vi "UT_TCP2Foxconn.vi"() -> ()   [LabVIEW 2019, in "TCP2Foxconn.lvlib"]
uses:
  TCP2Foxconn.lvlib
panel:
  in  "One shot Second HandShake":bool
  in  "One shot First HandShake":bool
  out "Second Handshake Response":string="NG;;ORA-06502: PL/SQL: numeric or value error: character to number conversion error\nORA-06512: at \"SFIS1.LASER_CARVING_AA\", line 34\n;SN:TKSR131A1T2222000031,OK,LASEREND;"
  out "First Handshake Response":string
  in  "Second HandShake":bool
  in  "First HandShake":bool
  in  "Result":string="OK"
  in  "Barcode":string="TKSR131A1T2222000031"
  out "Error Out":errorcluster
  in  "Error In":errorcluster
  in  "Close API":bool
  out "TCP connected":bool
  in  "Close Connection":bool
  in  "Open Connection":bool
  in  "IP address":string="10.61.39.233:60003"
  # "2111170002800000320754"
  # "TKSR131A1T2222000019"
  # "TKSR131A1T2222000031"
  # "TKSR131A1T2222000040"
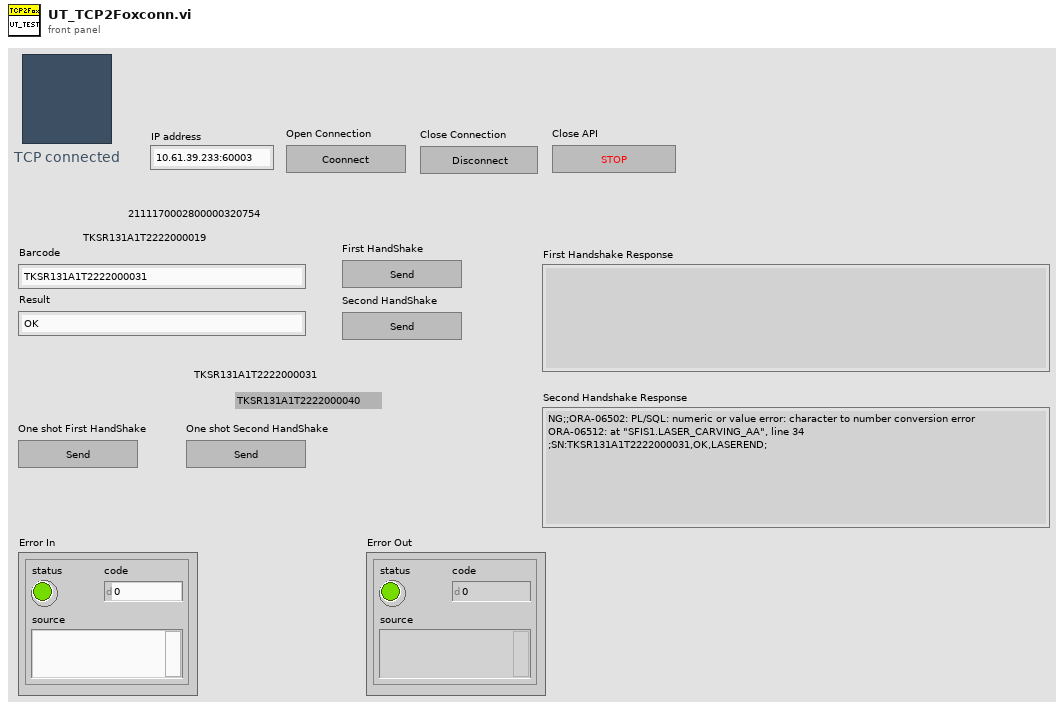
[diagram p1: front panel]
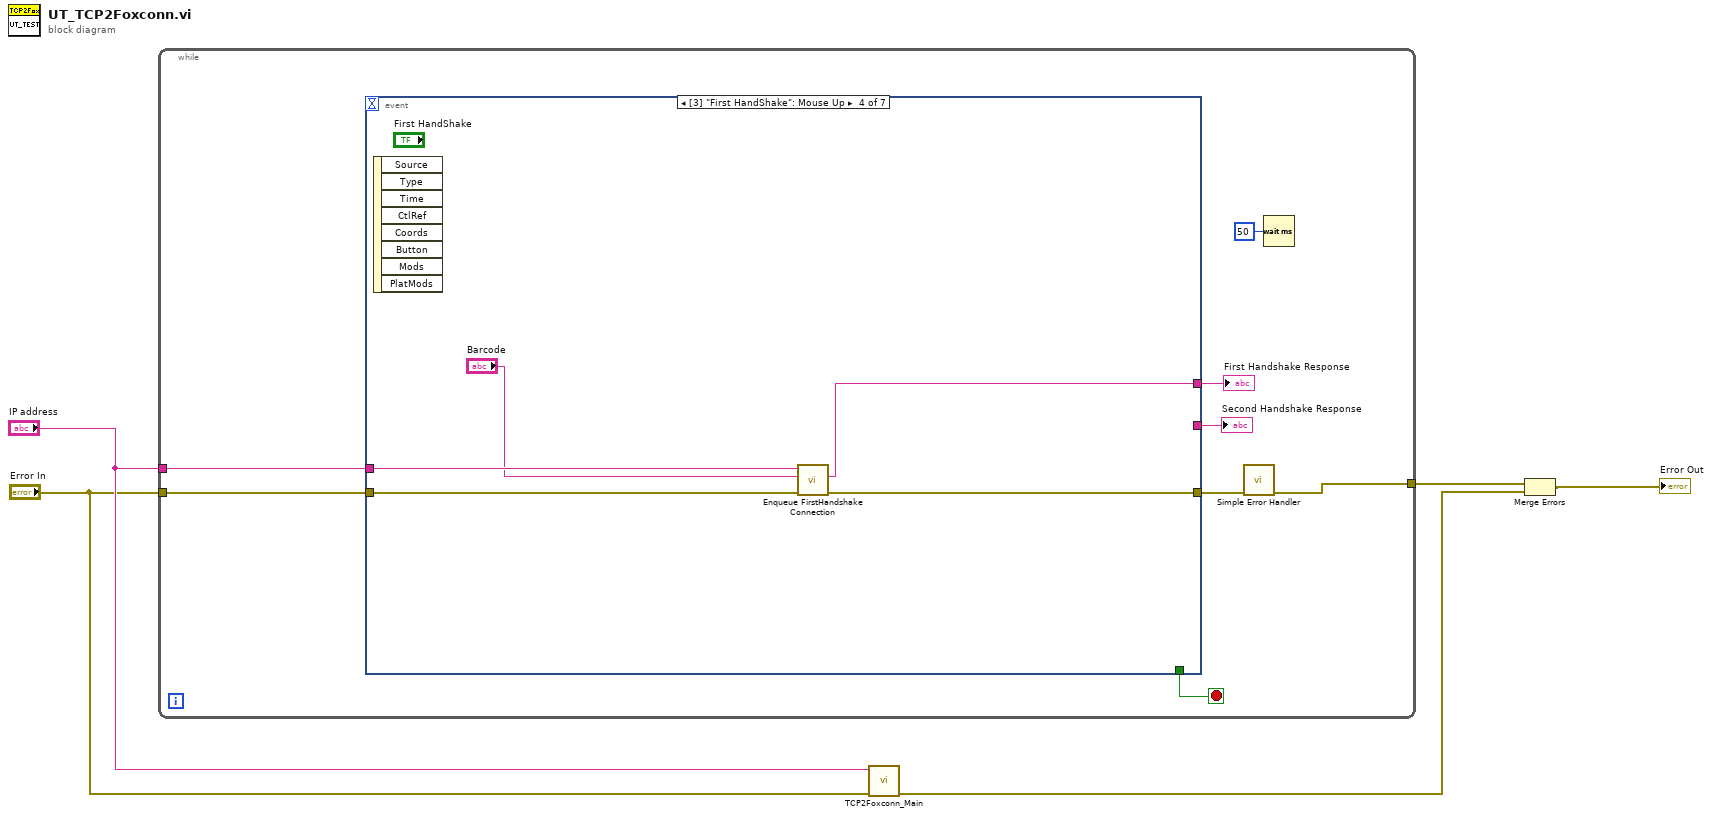
[diagram p0: block diagram]
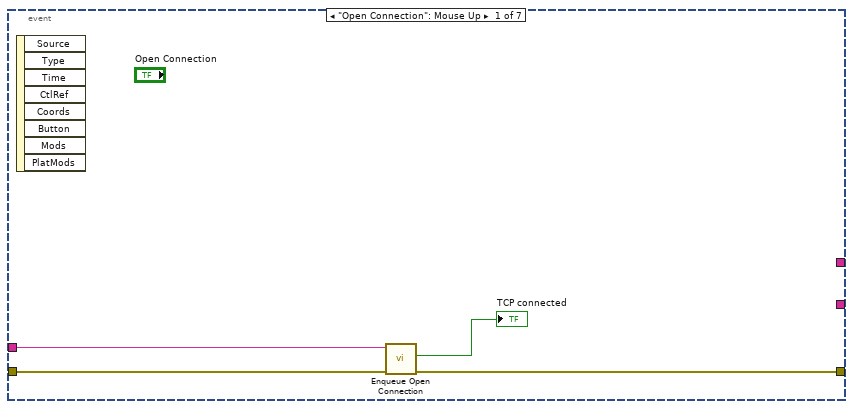
[diagram p2: hidden frame]
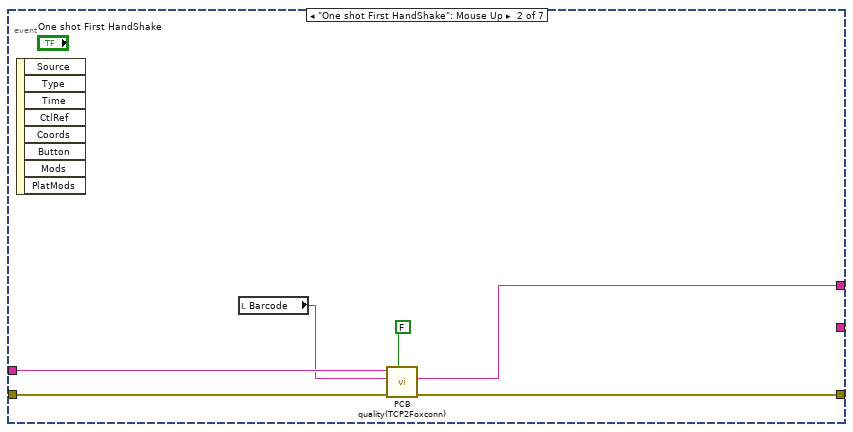
[diagram p3: hidden frame]
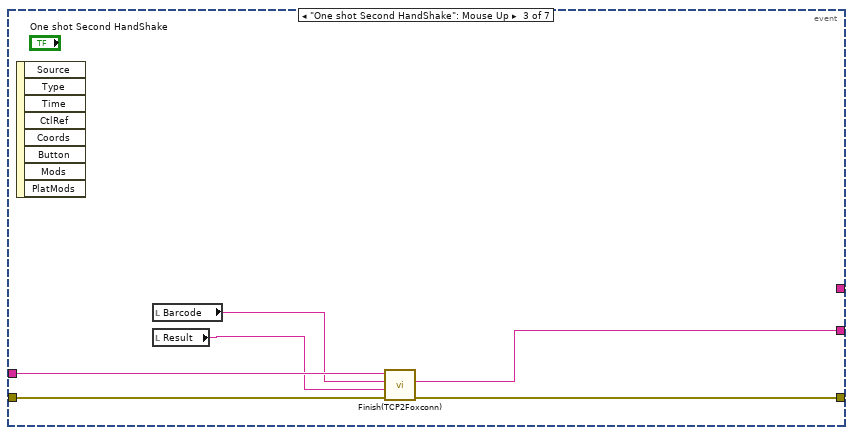
[diagram p4: hidden frame]
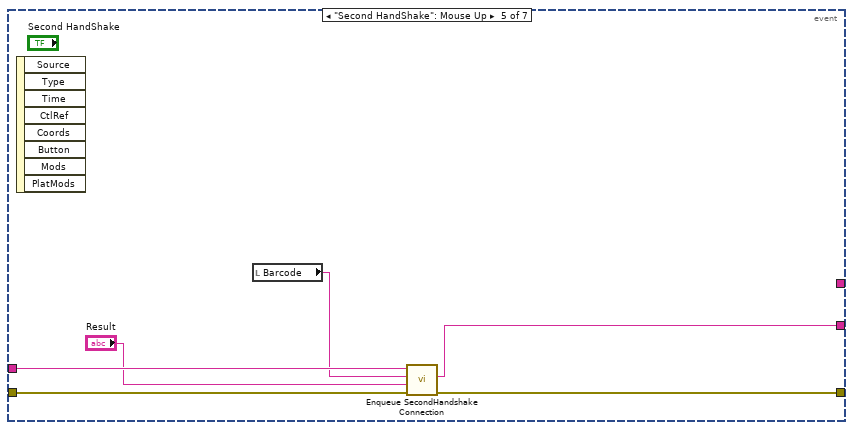
[diagram p5: hidden frame]
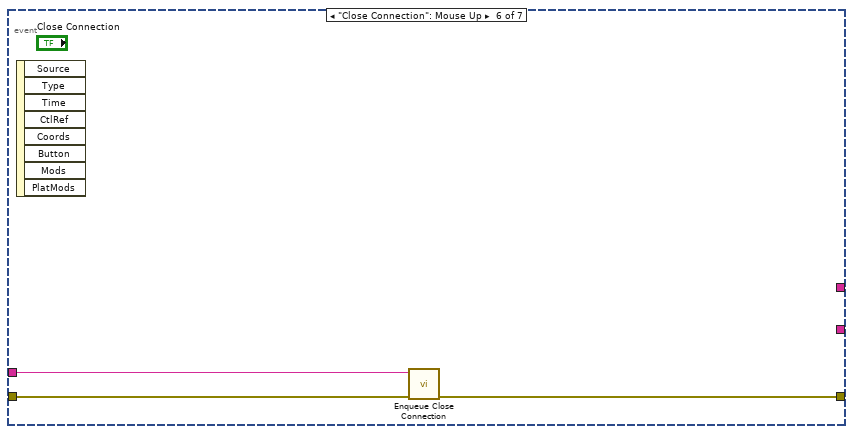
[diagram p6: hidden frame]
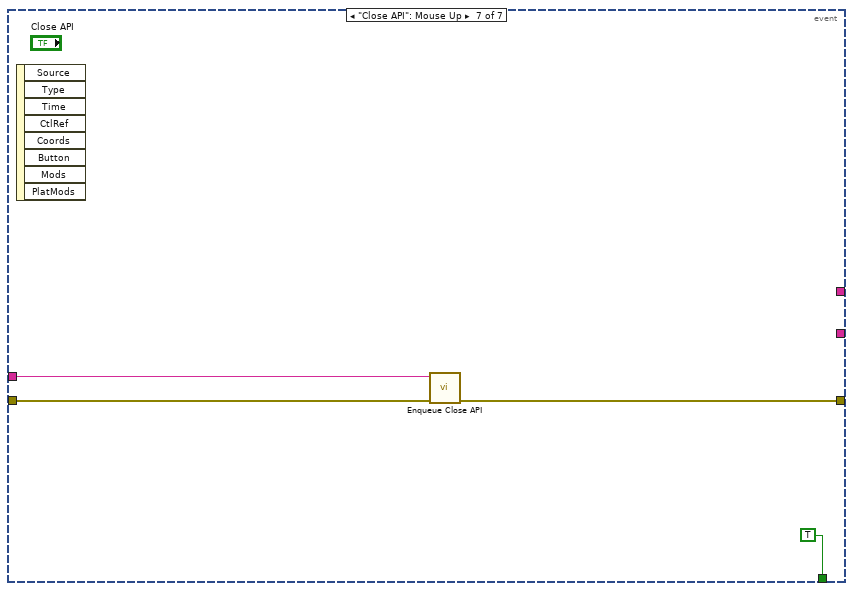
[diagram p7: hidden frame]
diagram:
  n1 = while {
    tunnel: "IP address" -> [w13]
    tunnel: "Error In" -> [w12]
    tunnel: [w10] -> w3
    stop <- w8 stop-if-true
    n2 = event shown="[3] \"First HandShake\": Mouse Up" {
      selector: _ -> [_ _ _ _ _ _ _]
      dyn-events: _ -> [_ _ _ _ _ _ _]
      timeout: _ -> [_ _ _ _ _ _ _]
      tunnel: w13 -> [w17 w23 w29 w34 w38 w41 w45]
      tunnel: w12 -> [w16 w22 w28 w33 w40 w43 w47]
      tunnel: [w15 w20 w24 w32 w39 w42 w46] -> w11
      tunnel: [_ _ _ _ _ _ TRUE] -> w8
      tunnel: [_ w21 _ w31 _ _ _] -> w7
      tunnel: [_ _ w25 _ w35 _ _] -> w6
      event "Open Connection": Mouse Up {
        n3 = event-data() -> ()  [unwired: 1 in, 8 out]
        n4 = call "Enqueue Open Connection.vi"("Error In"=w16, "Name"=w17) -> ("Error Out"=w15:errorcluster, "Connect?"=→"TCP connected":bool)  [unwired: 8 in]
      }
      event "One shot First HandShake": Mouse Up {
        n5 = event-data() -> ()  [unwired: 1 in, 8 out]
        n6 = local read "Barcode"() -> (w18:string)
        n7 = call "PCB quality(TCP2Foxconn).vi"("Bypass查詢"=FALSE, "error in (no error)"=w22, "Barcode"=w18, "TCP2Foxc"=w23) -> ("error out"=w20:errorcluster, "result"=w21:string)  [unwired: 6 in]
      }
      event "One shot Second HandShake": Mouse Up {
        n8 = event-data() -> ()  [unwired: 1 in, 8 out]
        n9 = local read "Barcode"() -> (w27:string)
        n10 = local read "Result"() -> (w26:string)
        n11 = call "Finish(TCP2Foxconn).vi"("error in (no error)"=w28, "Result"=w26, "Barcode"=w27, "TCP2Foxc"=w29) -> ("error out"=w24:errorcluster, "result"=w25:string)  [unwired: 6 in]
      }
      event "First HandShake": Mouse Up {
        n12 = event-data() -> ()  [unwired: 1 in, 8 out]
        n13 = call "Enqueue FirstHandshake Connection.vi"("Error In"=w33, "Barcode"="Barcode", "Name"=w34) -> ("Error Out"=w32:errorcluster, "Result"=w31:string)  [unwired: 7 in]
      }
      event "Second HandShake": Mouse Up {
        n14 = event-data() -> ()  [unwired: 1 in, 8 out]
        n15 = local read "Barcode"() -> (w36:string)
        n16 = call "Enqueue SecondHandshake Connection.vi"("Error In"=w40, "Result"="Result", "Barcode"=w36, "Name"=w38) -> ("Error Out"=w39:errorcluster, "Result"=w35:string)  [unwired: 6 in]
      }
      event "Close Connection": Mouse Up {
        n17 = event-data() -> ()  [unwired: 1 in, 8 out]
        n18 = call "Enqueue Close Connection.vi"("Error In"=w43, "Name"=w41) -> ("Error Out"=w42:errorcluster)  [unwired: 9 in]
      }
      event "Close API": Mouse Up {
        n19 = event-data() -> ()  [unwired: 1 in, 8 out]
        n20 = call "Enqueue Close API.vi"("Error In"=w47, "Name"=w45) -> ("Error Out"=w46:errorcluster)  [unwired: 9 in]
      }
    }
    "First Handshake Response" <- w7
    "Second Handshake Response" <- w6
    n21 = call <vilib>:"Simple Error Handler.vi"("error in (no error)"=w11) -> ("error out"=w10:errorcluster)  [unwired: 4 in, 4 out]
    n22 = Wait (ms)(milliseconds to wait=u32 50) -> ()  [unwired: 1 out]
  }
  n23 = call "TCP2Foxconn_Main.vi"("Error In"="Error In", "Name"="IP address") -> ("Error Out"=w2:errorcluster)  [unwired: 9 in]
  n24 = Merge Errors(w3, w2) -> (→"Error Out":errorcluster)
